vi "RDS Child Receive Message.vi"(8 "error in (no error)":errorcluster, 10 "RDS Message":refnum<class "RDS Message.lvclass">, 11 "Compass Instrument in":refnum<class "Compass Instrument.lvclass">) -> (0 "error out":errorcluster, 3 "Compass Instrument out":refnum<class "Compass Instrument.lvclass">)   [LabVIEW 2015, in "Compass Instrument.lvlib" / "Compass Instrument.lvclass"]
uses:
  Compass Instrument.lvclass
  RDS Framework/RDS Message Class/RDS Message.lvclass
  RDS Framework/RDS Message Class/RDS Message.lvclass/RDS Message.ctl
  RDS Child Messages/Compass/Set Mag Dev Message.lvclass
  RDS Child Messages/Compass/Set Mag Dev Message.lvclass/Set Mag Dev Message.ctl
  Compass Instrument.lvclass/Compass Instrument.ctl
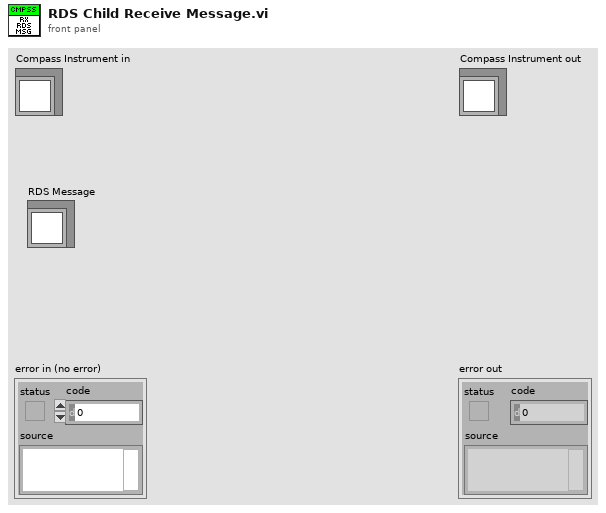
[diagram p1: front panel]
types:
  T1 = typedef "RDS Child Messages.lvlib/RDS Message ID.ctl" = enum16{"RDS Hello World", "String Message", "AIP_Status", "AIP_Command", "GPS_Data", "MCB_Command", "MCB_Status", "Compass_Data", "Depth_Data", "Battery_Data", "Contoller_State", "Set_Mag_Dev", "BTB_Shutdown", "State_Sample_Request", "State_Sample", "PID_Gains_Set", "Helm_Limiter_Set", "Helm_Heading_Command", "Helm_Steering_Command", "Helm_Status", "Controller_Message", "AIP_Set_Min_Depth", "Mission_Controller_State", "Mission_Upload", "Mission_Set_Op_and_Run", "Mission_Settings_Set"}
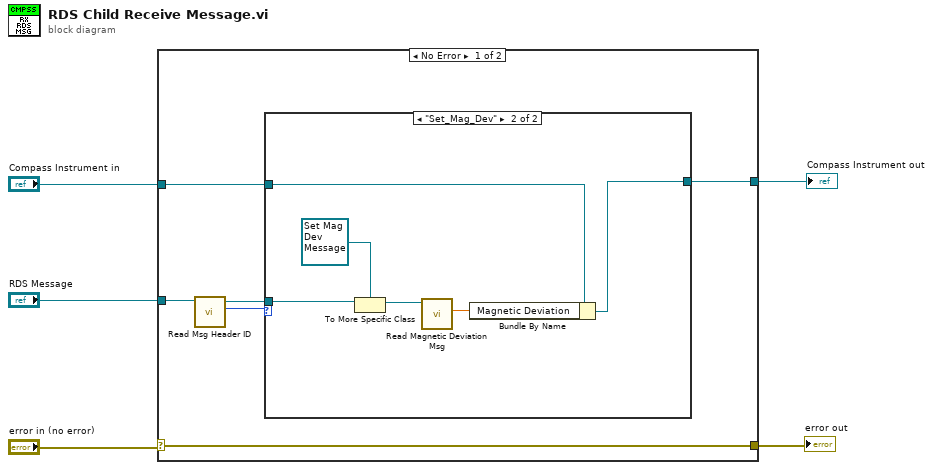
[diagram p0: block diagram]
diagram:
  n1 = case shown="No Error" "error in (no error)" {
    selector: "error in (no error)" -> [w11 w20]
    tunnel: [w11 w20] -> w5
    tunnel: "RDS Message" -> [w10 _]
    tunnel: "Compass Instrument in" -> [w7 w19]
    tunnel: [w6 w19] -> w1
    frame No Error {
      n2 = call "Read Msg Header ID.vi"("RDS Message in"=w10) -> ("Msg ID"=w9:T1, "RDS Message out"=w8:refnum<class "RDS Message.lvclass">)  [unwired: 6 in, 3 out]
      n3 = case shown="\"Set_Mag_Dev\"" w9 {
        tunnel: w8 -> [_ w17]
        tunnel: w7 -> [w12 w14]
        tunnel: [w12 w13] -> w6
        frame "RDS Hello World", Default {
        }
        frame "Set_Mag_Dev" {
          n4 = To More Specific Class(target class=refnum<class "Set Mag Dev Message.lvclass"> refnum ("RDS Child Messages.lvlib:Set Mag Dev Message.lvclass"), reference=w17) -> (specific class reference=w16:refnum<class "Set Mag Dev Message.lvclass">)  [unwired: 1 in, 1 out]
          n5 = call "Read Magnetic Deviation Msg.vi"("Set Mag Dev Message in"=w16) -> ("Magnetic Deviation"=w15:dbl)  [unwired: 8 in, 2 out]
          n6 = Bundle By Name(cluster=w14, "Magnetic Deviation"=w15) -> (w13:refnum<class "Compass Instrument.lvclass">)
        }
      }
    }
    frame Error {
    }
  }
  "error out" <- w5
  "Compass Instrument out" <- w1
